vi "VisualizePurePursuit.vi"(7 "Lookahead Point":cluster{dbl, dbl}, 8 "Robot":cluster{"Location":cluster{dbl, dbl}, dbl}, 9 "Lookahead":dbl, 10 "Curvature":dbl, 11 "Path":cluster{"x":dbl, "y":dbl}[](array[cluster])=[{"x"=0.0, "y"=10.0}, {"x"=0.0, "y"=80.0}, {"x"=75.0, "y"=125.0}, {"x"=120.0, "y"=125.0}, {"x"=150.0, "y"=50.0}]) -> (3 "Graph":cluster{cluster{"x":dbl, "y":dbl}[]}[](graph)=[{[{"x"=0.0, "y"=10.0}, {"x"=3.061616997868383e-17, "y"=10.5}, {"x"=6.123233995736766e-17, "y"=11.0}, {"x"=9.184850993605148e-17, "y"=11.5}, {"x"=1.2246467991473532e-16, "y"=12.0}, {"x"=1.5308084989341916e-16, "y"=12.5}, {"x"=1.8369701987210297e-16, "y"=13.0}, {"x"=2.143131898507868e-16, "y"=13.5}, {"x"=2.4492935982947064e-16, "y"=14.0}, {"x"=2.755455298081545e-16, "y"=14.5}, {"x"=3.061616997868383e-16, "y"=15.0}, {"x"=3.3677786976552215e-16, "y"=15.5}, {"x"=3.6739403974420594e-16, "y"=16.0}, {"x"=3.9801020972288977e-16, "y"=16.5}, {"x"=4.286263797015736e-16, "y"=17.0}, {"x"=4.592425496802575e-16, "y"=17.5}, {"x"=4.898587196589413e-16, "y"=18.0}, {"x"=5.204748896376251e-16, "y"=18.5}, {"x"=5.51091059616309e-16, "y"=19.0}, {"x"=5.817072295949927e-16, "y"=19.5}, {"x"=6.123233995736766e-16, "y"=20.0}, {"x"=6.429395695523604e-16, "y"=20.5}, {"x"=6.735557395310443e-16, "y"=21.0}, {"x"=7.041719095097281e-16, "y"=21.5}, {"x"=7.347880794884119e-16, "y"=22.0}, {"x"=7.654042494670958e-16, "y"=22.5}, {"x"=7.960204194457795e-16, "y"=23.0}, {"x"=8.266365894244634e-16, "y"=23.5}, {"x"=8.572527594031472e-16, "y"=24.0}, {"x"=8.878689293818311e-16, "y"=24.5}, {"x"=9.18485099360515e-16, "y"=25.0}, {"x"=9.491012693391988e-16, "y"=25.5}, {"x"=9.797174393178826e-16, "y"=26.0}, {"x"=1.0103336092965664e-15, "y"=26.5}, {"x"=1.0409497792752501e-15, "y"=27.0}, {"x"=1.0715659492539341e-15, "y"=27.5}, {"x"=1.102182119232618e-15, "y"=28.0}, {"x"=1.1327982892113017e-15, "y"=28.5}, {"x"=1.1634144591899855e-15, "y"=29.0}, {"x"=1.1940306291686695e-15, "y"=29.5}, {"x"=1.2246467991473533e-15, "y"=30.0}, {"x"=1.255262969126037e-15, "y"=30.5}, {"x"=1.2858791391047208e-15, "y"=31.0}, {"x"=1.3164953090834046e-15, "y"=31.5}, {"x"=1.3471114790620886e-15, "y"=32.0}, {"x"=1.3777276490407724e-15, "y"=32.5}, {"x"=1.4083438190194562e-15, "y"=33.0}, {"x"=1.43895998899814e-15, "y"=33.5}, {"x"=1.4695761589768238e-15, "y"=34.0}, {"x"=1.5001923289555077e-15, "y"=34.5}, {"x"=1.5308084989341915e-15, "y"=35.0}, {"x"=1.5614246689128753e-15, "y"=35.5}, {"x"=1.592040838891559e-15, "y"=36.0}, {"x"=1.622657008870243e-15, "y"=36.5}, {"x"=1.6532731788489269e-15, "y"=37.0}, {"x"=1.6838893488276107e-15, "y"=37.5}, {"x"=1.7145055188062944e-15, "y"=38.0}, {"x"=1.7451216887849782e-15, "y"=38.5}, {"x"=1.7757378587636622e-15, "y"=39.0}, {"x"=1.8063540287423458e-15, "y"=39.5}, {"x"=1.83697019872103e-15, "y"=40.0}, {"x"=1.8675863686997138e-15, "y"=40.5}, {"x"=1.8982025386783976e-15, "y"=41.0}, {"x"=1.9288187086570813e-15, "y"=41.5}, {"x"=1.959434878635765e-15, "y"=42.0}, {"x"=1.990051048614449e-15, "y"=42.5}, {"x"=2.0206672185931327e-15, "y"=43.0}, {"x"=2.0512833885718165e-15, "y"=43.5}, {"x"=2.0818995585505003e-15, "y"=44.0}, {"x"=2.1125157285291845e-15, "y"=44.5}, {"x"=2.1431318985078682e-15, "y"=45.0}, {"x"=2.173748068486552e-15, "y"=45.5}, {"x"=2.204364238465236e-15, "y"=46.0}, {"x"=2.2349804084439196e-15, "y"=46.5}, {"x"=2.2655965784226034e-15, "y"=47.0}, {"x"=2.296212748401287e-15, "y"=47.5}, {"x"=2.326828918379971e-15, "y"=48.0}, {"x"=2.3574450883586548e-15, "y"=48.5}, {"x"=2.388061258337339e-15, "y"=49.0}, {"x"=2.4186774283160227e-15, "y"=49.5}, {"x"=2.4492935982947065e-15, "y"=50.0}, {"x"=2.4799097682733903e-15, "y"=50.5}, {"x"=2.510525938252074e-15, "y"=51.0}, {"x"=2.541142108230758e-15, "y"=51.5}, {"x"=2.5717582782094417e-15, "y"=52.0}, {"x"=2.6023744481881254e-15, "y"=52.5}, {"x"=2.6329906181668092e-15, "y"=53.0}, {"x"=2.6636067881454934e-15, "y"=53.5}, {"x"=2.6942229581241772e-15, "y"=54.0}, {"x"=2.724839128102861e-15, "y"=54.5}, {"x"=2.7554552980815448e-15, "y"=55.0}, {"x"=2.7860714680602286e-15, "y"=55.5}, {"x"=2.8166876380389124e-15, "y"=56.0}, {"x"=2.847303808017596e-15, "y"=56.5}, {"x"=2.87791997799628e-15, "y"=57.0}, {"x"=2.9085361479749637e-15, "y"=57.5}, {"x"=2.9391523179536475e-15, "y"=58.0}, {"x"=2.9697684879323317e-15, "y"=58.5}, {"x"=3.0003846579110155e-15, "y"=59.0}, {"x"=3.0310008278896993e-15, "y"=59.5}, {"x"=3.061616997868383e-15, "y"=60.0}, {"x"=3.092233167847067e-15, "y"=60.5}, {"x"=3.1228493378257506e-15, "y"=61.0}, {"x"=3.1534655078044344e-15, "y"=61.5}, {"x"=3.184081677783118e-15, "y"=62.0}, {"x"=3.214697847761802e-15, "y"=62.5}, {"x"=3.245314017740486e-15, "y"=63.0}, {"x"=3.27593018771917e-15, "y"=63.5}, {"x"=3.3065463576978537e-15, "y"=64.0}, {"x"=3.3371625276765375e-15, "y"=64.5}, {"x"=3.3677786976552213e-15, "y"=65.0}, {"x"=3.398394867633905e-15, "y"=65.5}, {"x"=3.429011037612589e-15, "y"=66.0}, {"x"=3.4596272075912727e-15, "y"=66.5}, {"x"=3.4902433775699565e-15, "y"=67.0}, {"x"=3.5208595475486406e-15, "y"=67.5}, {"x"=3.5514757175273244e-15, "y"=68.0}, {"x"=3.582091887506008e-15, "y"=68.5}, {"x"=3.6127080574846916e-15, "y"=69.0}, {"x"=3.643324227463376e-15, "y"=69.5}, {"x"=3.67394039744206e-15, "y"=70.0}, {"x"=3.704556567420744e-15, "y"=70.5}, {"x"=3.7351727373994275e-15, "y"=71.0}, {"x"=3.765788907378111e-15, "y"=71.5}, {"x"=3.796405077356795e-15, "y"=72.0}, {"x"=3.827021247335479e-15, "y"=72.5}, {"x"=3.857637417314163e-15, "y"=73.0}, {"x"=3.8882535872928465e-15, "y"=73.5}, {"x"=3.91886975727153e-15, "y"=74.0}, {"x"=3.949485927250214e-15, "y"=74.5}, {"x"=3.980102097228898e-15, "y"=75.0}, {"x"=4.010718267207582e-15, "y"=75.5}, {"x"=4.0413344371862654e-15, "y"=76.0}, {"x"=4.071950607164949e-15, "y"=76.5}, {"x"=4.102566777143633e-15, "y"=77.0}, {"x"=4.133182947122317e-15, "y"=77.5}, {"x"=4.1637991171010006e-15, "y"=78.0}, {"x"=4.194415287079684e-15, "y"=78.5}, {"x"=4.225031457058369e-15, "y"=79.0}, {"x"=4.255647627037053e-15, "y"=79.5}, {"x"=0.0, "y"=80.0}, {"x"=0.4287464628562721, "y"=80.25724787771377}, {"x"=0.8574929257125442, "y"=80.51449575542753}, {"x"=1.2862393885688164, "y"=80.77174363314128}, {"x"=1.7149858514250884, "y"=81.02899151085505}, {"x"=2.1437323142813605, "y"=81.28623938856882}, {"x"=2.5724787771376327, "y"=81.54348726628258}, {"x"=3.0012252399939046, "y"=81.80073514399635}, {"x"=3.429971702850177, "y"=82.0579830217101}, {"x"=3.858718165706449, "y"=82.31523089942387}, {"x"=4.287464628562721, "y"=82.57247877713763}, {"x"=4.716211091418993, "y"=82.8297266548514}, {"x"=5.1449575542752655, "y"=83.08697453256516}, {"x"=5.573704017131537, "y"=83.34422241027892}, {"x"=6.002450479987809, "y"=83.60147028799268}, {"x"=6.431196942844082, "y"=83.85871816570645}, {"x"=6.859943405700354, "y"=84.11596604342022}, {"x"=7.2886898685566255, "y"=84.37321392113398}, {"x"=7.717436331412898, "y"=84.63046179884773}, {"x"=8.14618279426917, "y"=84.8877096765615}, {"x"=8.574929257125442, "y"=85.14495755427527}, {"x"=9.003675719981715, "y"=85.40220543198903}, {"x"=9.432422182837986, "y"=85.6594533097028}, {"x"=9.861168645694258, "y"=85.91670118741655}, {"x"=10.289915108550531, "y"=86.17394906513032}, {"x"=10.718661571406802, "y"=86.43119694284408}, {"x"=11.147408034263075, "y"=86.68844482055785}, {"x"=11.576154497119347, "y"=86.94569269827161}, {"x"=12.004900959975618, "y"=87.20294057598537}, {"x"=12.433647422831891, "y"=87.46018845369913}, {"x"=12.862393885688164, "y"=87.7174363314129}, {"x"=13.291140348544435, "y"=87.97468420912666}, {"x"=13.719886811400707, "y"=88.23193208684043}, {"x"=14.14863327425698, "y"=88.48917996455418}, {"x"=14.577379737113251, "y"=88.74642784226795}, {"x"=15.006126199969524, "y"=89.00367571998171}, {"x"=15.434872662825796, "y"=89.26092359769548}, {"x"=15.863619125682067, "y"=89.51817147540925}, {"x"=16.29236558853834, "y"=89.775419353123}, {"x"=16.721112051394613, "y"=90.03266723083676}, {"x"=17.149858514250884, "y"=90.28991510855053}, {"x"=17.578604977107155, "y"=90.5471629862643}, {"x"=18.00735143996343, "y"=90.80441086397806}, {"x"=18.4360979028197, "y"=91.06165874169182}, {"x"=18.86484436567597, "y"=91.31890661940558}, {"x"=19.293590828532245, "y"=91.57615449711935}, {"x"=19.722337291388516, "y"=91.83340237483311}, {"x"=20.151083754244787, "y"=92.09065025254688}, {"x"=20.579830217101062, "y"=92.34789813026063}, {"x"=21.008576679957333, "y"=92.6051460079744}, {"x"=21.437323142813604, "y"=92.86239388568816}, {"x"=21.86606960566988, "y"=93.11964176340193}, {"x"=22.29481606852615, "y"=93.3768896411157}, {"x"=22.72356253138242, "y"=93.63413751882945}, {"x"=23.152308994238695, "y"=93.89138539654321}, {"x"=23.581055457094966, "y"=94.14863327425698}, {"x"=24.009801919951236, "y"=94.40588115197075}, {"x"=24.43854838280751, "y"=94.66312902968451}, {"x"=24.867294845663782, "y"=94.92037690739826}, {"x"=25.296041308520053, "y"=95.17762478511203}, {"x"=25.724787771376327, "y"=95.4348726628258}, {"x"=26.1535342342326, "y"=95.69212054053956}, {"x"=26.58228069708887, "y"=95.94936841825333}, {"x"=27.011027159945144, "y"=96.20661629596708}, {"x"=27.439773622801415, "y"=96.46386417368085}, {"x"=27.868520085657686, "y"=96.72111205139461}, {"x"=28.29726654851396, "y"=96.97835992910838}, {"x"=28.72601301137023, "y"=97.23560780682214}, {"x"=29.154759474226502, "y"=97.4928556845359}, {"x"=29.583505937082776, "y"=97.75010356224966}, {"x"=30.012252399939047, "y"=98.00735143996343}, {"x"=30.44099886279532, "y"=98.2645993176772}, {"x"=30.869745325651593, "y"=98.52184719539096}, {"x"=31.298491788507864, "y"=98.77909507310471}, {"x"=31.727238251364135, "y"=99.03634295081848}, {"x"=32.15598471422041, "y"=99.29359082853225}, {"x"=32.58473117707668, "y"=99.55083870624601}, {"x"=33.01347763993295, "y"=99.80808658395978}, {"x"=33.442224102789226, "y"=100.06533446167353}, {"x"=33.87097056564549, "y"=100.3225823393873}, {"x"=34.29971702850177, "y"=100.57983021710106}, {"x"=34.72846349135804, "y"=100.83707809481483}, {"x"=35.15720995421431, "y"=101.0943259725286}, {"x"=35.585956417070584, "y"=101.35157385024235}, {"x"=36.01470287992686, "y"=101.60882172795611}, {"x"=36.443449342783126, "y"=101.86606960566988}, {"x"=36.8721958056394, "y"=102.12331748338364}, {"x"=37.300942268495675, "y"=102.38056536109741}, {"x"=37.72968873135194, "y"=102.63781323881116}, {"x"=38.15843519420822, "y"=102.89506111652493}, {"x"=38.58718165706449, "y"=103.1523089942387}, {"x"=39.01592811992076, "y"=103.40955687195246}, {"x"=39.44467458277703, "y"=103.66680474966623}, {"x"=39.87342104563331, "y"=103.92405262737998}, {"x"=40.302167508489575, "y"=104.18130050509374}, {"x"=40.73091397134585, "y"=104.43854838280751}, {"x"=41.159660434202124, "y"=104.69579626052128}, {"x"=41.58840689705839, "y"=104.95304413823504}, {"x"=42.017153359914666, "y"=105.2102920159488}, {"x"=42.44589982277094, "y"=105.46753989366256}, {"x"=42.87464628562721, "y"=105.72478777137633}, {"x"=43.30339274848348, "y"=105.9820356490901}, {"x"=43.73213921133976, "y"=106.23928352680386}, {"x"=44.160885674196024, "y"=106.49653140451761}, {"x"=44.5896321370523, "y"=106.75377928223138}, {"x"=45.01837859990857, "y"=107.01102715994514}, {"x"=45.44712506276484, "y"=107.26827503765891}, {"x"=45.875871525621115, "y"=107.52552291537268}, {"x"=46.30461798847739, "y"=107.78277079308643}, {"x"=46.73336445133366, "y"=108.0400186708002}, {"x"=47.16211091418993, "y"=108.29726654851396}, {"x"=47.590857377046206, "y"=108.55451442622773}, {"x"=48.01960383990247, "y"=108.81176230394149}, {"x"=48.44835030275875, "y"=109.06901018165524}, {"x"=48.87709676561502, "y"=109.32625805936901}, {"x"=49.30584322847129, "y"=109.58350593708278}, {"x"=49.734589691327564, "y"=109.84075381479654}, {"x"=50.16333615418384, "y"=110.09800169251031}, {"x"=50.592082617040106, "y"=110.35524957022406}, {"x"=51.02082907989638, "y"=110.61249744793783}, {"x"=51.449575542752655, "y"=110.86974532565159}, {"x"=51.87832200560892, "y"=111.12699320336536}, {"x"=52.3070684684652, "y"=111.38424108107913}, {"x"=52.73581493132147, "y"=111.64148895879288}, {"x"=53.16456139417774, "y"=111.89873683650664}, {"x"=53.59330785703401, "y"=112.15598471422041}, {"x"=54.02205431989029, "y"=112.41323259193418}, {"x"=54.450800782746555, "y"=112.67048046964794}, {"x"=54.87954724560283, "y"=112.9277283473617}, {"x"=55.308293708459104, "y"=113.18497622507547}, {"x"=55.73704017131537, "y"=113.44222410278923}, {"x"=56.165786634171646, "y"=113.69947198050299}, {"x"=56.59453309702792, "y"=113.95671985821676}, {"x"=57.02327955988419, "y"=114.21396773593051}, {"x"=57.45202602274046, "y"=114.47121561364429}, {"x"=57.88077248559674, "y"=114.72846349135804}, {"x"=58.309518948453004, "y"=114.98571136907181}, {"x"=58.73826541130928, "y"=115.24295924678557}, {"x"=59.16701187416555, "y"=115.50020712449933}, {"x"=59.59575833702182, "y"=115.7574550022131}, {"x"=60.024504799878095, "y"=116.01470287992686}, {"x"=60.45325126273437, "y"=116.27195075764062}, {"x"=60.88199772559064, "y"=116.52919863535439}, {"x"=61.31074418844691, "y"=116.78644651306814}, {"x"=61.739490651303186, "y"=117.04369439078192}, {"x"=62.16823711415945, "y"=117.30094226849567}, {"x"=62.59698357701573, "y"=117.55819014620944}, {"x"=63.025730039872, "y"=117.8154380239232}, {"x"=63.45447650272827, "y"=118.07268590163696}, {"x"=63.883222965584544, "y"=118.32993377935074}, {"x"=64.31196942844082, "y"=118.58718165706449}, {"x"=64.74071589129709, "y"=118.84442953477826}, {"x"=65.16946235415335, "y"=119.10167741249202}, {"x"=65.59820881700963, "y"=119.35892529020578}, {"x"=66.0269552798659, "y"=119.61617316791956}, {"x"=66.45570174272217, "y"=119.87342104563331}, {"x"=66.88444820557845, "y"=120.13066892334707}, {"x"=67.31319466843472, "y"=120.38791680106084}, {"x"=67.74194113129099, "y"=120.64516467877459}, {"x"=68.17068759414727, "y"=120.90241255648837}, {"x"=68.59943405700353, "y"=121.15966043420212}, {"x"=69.0281805198598, "y"=121.41690831191589}, {"x"=69.45692698271608, "y"=121.67415618962966}, {"x"=69.88567344557235, "y"=121.93140406734341}, {"x"=70.31441990842862, "y"=122.18865194505719}, {"x"=70.7431663712849, "y"=122.44589982277094}, {"x"=71.17191283414117, "y"=122.7031477004847}, {"x"=71.60065929699743, "y"=122.96039557819847}, {"x"=72.02940575985372, "y"=123.21764345591222}, {"x"=72.45815222270998, "y"=123.474891333626}, {"x"=72.88689868556625, "y"=123.73213921133976}, {"x"=73.31564514842253, "y"=123.98938708905352}, {"x"=73.7443916112788, "y"=124.24663496676729}, {"x"=74.17313807413507, "y"=124.50388284448104}, {"x"=74.60188453699135, "y"=124.76113072219482}, {"x"=75.0, "y"=125.0}, {"x"=75.5, "y"=125.0}, {"x"=76.0, "y"=125.0}, {"x"=76.5, "y"=125.0}, {"x"=77.0, "y"=125.0}, {"x"=77.5, "y"=125.0}, {"x"=78.0, "y"=125.0}, {"x"=78.5, "y"=125.0}, {"x"=79.0, "y"=125.0}, {"x"=79.5, "y"=125.0}, {"x"=80.0, "y"=125.0}, {"x"=80.5, "y"=125.0}, {"x"=81.0, "y"=125.0}, {"x"=81.5, "y"=125.0}, {"x"=82.0, "y"=125.0}, {"x"=82.5, "y"=125.0}, {"x"=83.0, "y"=125.0}, {"x"=83.5, "y"=125.0}, {"x"=84.0, "y"=125.0}, {"x"=84.5, "y"=125.0}, {"x"=85.0, "y"=125.0}, {"x"=85.5, "y"=125.0}, {"x"=86.0, "y"=125.0}, {"x"=86.5, "y"=125.0}, {"x"=87.0, "y"=125.0}, {"x"=87.5, "y"=125.0}, {"x"=88.0, "y"=125.0}, {"x"=88.5, "y"=125.0}, {"x"=89.0, "y"=125.0}, {"x"=89.5, "y"=125.0}, {"x"=90.0, "y"=125.0}, {"x"=90.5, "y"=125.0}, {"x"=91.0, "y"=125.0}, {"x"=91.5, "y"=125.0}, {"x"=92.0, "y"=125.0}, {"x"=92.5, "y"=125.0}, {"x"=93.0, "y"=125.0}, {"x"=93.5, "y"=125.0}, {"x"=94.0, "y"=125.0}, {"x"=94.5, "y"=125.0}, {"x"=95.0, "y"=125.0}, {"x"=95.5, "y"=125.0}, {"x"=96.0, "y"=125.0}, {"x"=96.5, "y"=125.0}, {"x"=97.0, "y"=125.0}, {"x"=97.5, "y"=125.0}, {"x"=98.0, "y"=125.0}, {"x"=98.5, "y"=125.0}, {"x"=99.0, "y"=125.0}, {"x"=99.5, "y"=125.0}, {"x"=100.0, "y"=125.0}, {"x"=100.5, "y"=125.0}, {"x"=101.0, "y"=125.0}, {"x"=101.5, "y"=125.0}, {"x"=102.0, "y"=125.0}, {"x"=102.5, "y"=125.0}, {"x"=103.0, "y"=125.0}, {"x"=103.5, "y"=125.0}, {"x"=104.0, "y"=125.0}, {"x"=104.5, "y"=125.0}, {"x"=105.0, "y"=125.0}, {"x"=105.5, "y"=125.0}, {"x"=106.0, "y"=125.0}, {"x"=106.5, "y"=125.0}, {"x"=107.0, "y"=125.0}, {"x"=107.5, "y"=125.0}, {"x"=108.0, "y"=125.0}, {"x"=108.5, "y"=125.0}, {"x"=109.0, "y"=125.0}, {"x"=109.5, "y"=125.0}, {"x"=110.0, "y"=125.0}, {"x"=110.5, "y"=125.0}, {"x"=111.0, "y"=125.0}, {"x"=111.5, "y"=125.0}, {"x"=112.0, "y"=125.0}, {"x"=112.5, "y"=125.0}, {"x"=113.0, "y"=125.0}, {"x"=113.5, "y"=125.0}, {"x"=114.0, "y"=125.0}, {"x"=114.5, "y"=125.0}, {"x"=115.0, "y"=125.0}, {"x"=115.5, "y"=125.0}, {"x"=116.0, "y"=125.0}, {"x"=116.5, "y"=125.0}, {"x"=117.0, "y"=125.0}, {"x"=117.5, "y"=125.0}, {"x"=118.0, "y"=125.0}, {"x"=118.5, "y"=125.0}, {"x"=119.0, "y"=125.0}, {"x"=119.5, "y"=125.0}, {"x"=120.0, "y"=125.0}, {"x"=120.18569533817706, "y"=124.53576165455738}, {"x"=120.37139067635411, "y"=124.07152330911474}, {"x"=120.55708601453115, "y"=123.60728496367211}, {"x"=120.7427813527082, "y"=123.14304661822948}, {"x"=120.92847669088526, "y"=122.67880827278685}, {"x"=121.11417202906232, "y"=122.21456992734423}, {"x"=121.29986736723936, "y"=121.75033158190159}, {"x"=121.48556270541641, "y"=121.28609323645897}, {"x"=121.67125804359347, "y"=120.82185489101633}, {"x"=121.85695338177052, "y"=120.3576165455737}, {"x"=122.04264871994756, "y"=119.89337820013107}, {"x"=122.22834405812462, "y"=119.42913985468844}, {"x"=122.41403939630167, "y"=118.96490150924582}, {"x"=122.59973473447873, "y"=118.50066316380318}, {"x"=122.78543007265577, "y"=118.03642481836056}, {"x"=122.97112541083283, "y"=117.57218647291792}, {"x"=123.15682074900988, "y"=117.1079481274753}, {"x"=123.34251608718694, "y"=116.64370978203266}, {"x"=123.52821142536399, "y"=116.17947143659003}, {"x"=123.71390676354103, "y"=115.71523309114741}, {"x"=123.89960210171809, "y"=115.25099474570477}, {"x"=124.08529743989514, "y"=114.78675640026215}, {"x"=124.2709927780722, "y"=114.32251805481951}, {"x"=124.45668811624924, "y"=113.85827970937689}, {"x"=124.6423834544263, "y"=113.39404136393426}, {"x"=124.82807879260335, "y"=112.92980301849163}, {"x"=125.0137741307804, "y"=112.465564673049}, {"x"=125.19946946895746, "y"=112.00132632760636}, {"x"=125.3851648071345, "y"=111.53708798216374}, {"x"=125.57086014531156, "y"=111.07284963672112}, {"x"=125.75655548348861, "y"=110.60861129127848}, {"x"=125.94225082166567, "y"=110.14437294583585}, {"x"=126.12794615984271, "y"=109.68013460039322}, {"x"=126.31364149801976, "y"=109.2158962549506}, {"x"=126.49933683619682, "y"=108.75165790950797}, {"x"=126.68503217437387, "y"=108.28741956406533}, {"x"=126.87072751255091, "y"=107.82318121862271}, {"x"=127.05642285072797, "y"=107.35894287318007}, {"x"=127.24211818890502, "y"=106.89470452773745}, {"x"=127.42781352708208, "y"=106.43046618229482}, {"x"=127.61350886525912, "y"=105.96622783685218}, {"x"=127.79920420343618, "y"=105.50198949140955}, {"x"=127.98489954161323, "y"=105.03775114596692}, {"x"=128.1705948797903, "y"=104.5735128005243}, {"x"=128.35629021796734, "y"=104.10927445508166}, {"x"=128.5419855561444, "y"=103.64503610963904}, {"x"=128.72768089432145, "y"=103.1807977641964}, {"x"=128.91337623249848, "y"=102.71655941875377}, {"x"=129.09907157067553, "y"=102.25232107331115}, {"x"=129.2847669088526, "y"=101.78808272786851}, {"x"=129.47046224702964, "y"=101.32384438242589}, {"x"=129.6561575852067, "y"=100.85960603698325}, {"x"=129.84185292338375, "y"=100.39536769154063}, {"x"=130.0275482615608, "y"=99.931129346098}, {"x"=130.21324359973786, "y"=99.46689100065537}, {"x"=130.39893893791492, "y"=99.00265265521274}, {"x"=130.58463427609195, "y"=98.5384143097701}, {"x"=130.770329614269, "y"=98.07417596432748}, {"x"=130.95602495244606, "y"=97.60993761888486}, {"x"=131.1417202906231, "y"=97.14569927344222}, {"x"=131.32741562880017, "y"=96.6814609279996}, {"x"=131.51311096697722, "y"=96.21722258255696}, {"x"=131.69880630515428, "y"=95.75298423711433}, {"x"=131.88450164333133, "y"=95.28874589167171}, {"x"=132.07019698150836, "y"=94.82450754622907}, {"x"=132.25589231968542, "y"=94.36026920078645}, {"x"=132.44158765786247, "y"=93.89603085534381}, {"x"=132.62728299603953, "y"=93.43179250990119}, {"x"=132.81297833421658, "y"=92.96755416445856}, {"x"=132.99867367239364, "y"=92.50331581901592}, {"x"=133.1843690105707, "y"=92.03907747357329}, {"x"=133.37006434874775, "y"=91.57483912813066}, {"x"=133.55575968692477, "y"=91.11060078268804}, {"x"=133.74145502510183, "y"=90.64636243724541}, {"x"=133.92715036327888, "y"=90.18212409180278}, {"x"=134.11284570145594, "y"=89.71788574636014}, {"x"=134.298541039633, "y"=89.25364740091752}, {"x"=134.48423637781005, "y"=88.78940905547489}, {"x"=134.6699317159871, "y"=88.32517071003227}, {"x"=134.85562705416416, "y"=87.86093236458963}, {"x"=135.04132239234121, "y"=87.39669401914699}, {"x"=135.22701773051824, "y"=86.93245567370437}, {"x"=135.4127130686953, "y"=86.46821732826174}, {"x"=135.59840840687235, "y"=86.0039789828191}, {"x"=135.7841037450494, "y"=85.53974063737648}, {"x"=135.96979908322646, "y"=85.07550229193384}, {"x"=136.15549442140352, "y"=84.61126394649122}, {"x"=136.34118975958057, "y"=84.1470256010486}, {"x"=136.52688509775763, "y"=83.68278725560596}, {"x"=136.71258043593468, "y"=83.21854891016332}, {"x"=136.8982757741117, "y"=82.7543105647207}, {"x"=137.08397111228876, "y"=82.29007221927807}, {"x"=137.26966645046582, "y"=81.82583387383545}, {"x"=137.45536178864288, "y"=81.36159552839281}, {"x"=137.64105712681993, "y"=80.89735718295017}, {"x"=137.82675246499699, "y"=80.43311883750755}, {"x"=138.01244780317404, "y"=79.96888049206493}, {"x"=138.1981431413511, "y"=79.5046421466223}, {"x"=138.38383847952815, "y"=79.04040380117966}, {"x"=138.56953381770518, "y"=78.57616545573703}, {"x"=138.75522915588223, "y"=78.1119271102944}, {"x"=138.9409244940593, "y"=77.64768876485178}, {"x"=139.12661983223634, "y"=77.18345041940916}, {"x"=139.3123151704134, "y"=76.71921207396652}, {"x"=139.49801050859045, "y"=76.25497372852388}, {"x"=139.6837058467675, "y"=75.79073538308126}, {"x"=139.86940118494456, "y"=75.32649703763863}, {"x"=140.05509652312162, "y"=74.86225869219601}, {"x"=140.24079186129865, "y"=74.39802034675337}, {"x"=140.4264871994757, "y"=73.93378200131073}, {"x"=140.61218253765276, "y"=73.46954365586811}, {"x"=140.7978778758298, "y"=73.00530531042548}, {"x"=140.98357321400687, "y"=72.54106696498285}, {"x"=141.16926855218392, "y"=72.07682861954022}, {"x"=141.35496389036098, "y"=71.61259027409758}, {"x"=141.540659228538, "y"=71.14835192865496}, {"x"=141.72635456671506, "y"=70.68411358321234}, {"x"=141.91204990489211, "y"=70.2198752377697}, {"x"=142.09774524306917, "y"=69.75563689232706}, {"x"=142.28344058124623, "y"=69.29139854688444}, {"x"=142.46913591942328, "y"=68.82716020144181}, {"x"=142.65483125760034, "y"=68.36292185599919}, {"x"=142.8405265957774, "y"=67.89868351055655}, {"x"=143.02622193395445, "y"=67.43444516511391}, {"x"=143.21191727213147, "y"=66.97020681967129}, {"x"=143.39761261030853, "y"=66.50596847422867}, {"x"=143.58330794848558, "y"=66.04173012878604}, {"x"=143.76900328666264, "y"=65.5774917833434}, {"x"=143.9546986248397, "y"=65.11325343790077}, {"x"=144.14039396301675, "y"=64.64901509245814}, {"x"=144.3260893011938, "y"=64.18477674701552}, {"x"=144.51178463937086, "y"=63.72053840157289}, {"x"=144.6974799775479, "y"=63.25630005613026}, {"x"=144.88317531572494, "y"=62.792061710687626}, {"x"=145.068870653902, "y"=62.327823365244996}, {"x"=145.25456599207905, "y"=61.863585019802365}, {"x"=145.4402613302561, "y"=61.39934667435974}, {"x"=145.62595666843316, "y"=60.93510832891711}, {"x"=145.81165200661022, "y"=60.47086998347447}, {"x"=145.99734734478727, "y"=60.00663163803185}, {"x"=146.18304268296433, "y"=59.542393292589225}, {"x"=146.36873802114138, "y"=59.07815494714659}, {"x"=146.5544333593184, "y"=58.61391660170396}, {"x"=146.74012869749546, "y"=58.149678256261325}, {"x"=146.92582403567252, "y"=57.6854399108187}, {"x"=147.11151937384957, "y"=57.22120156537608}, {"x"=147.29721471202663, "y"=56.75696321993344}, {"x"=147.48291005020369, "y"=56.292724874490816}, {"x"=147.66860538838074, "y"=55.82848652904818}, {"x"=147.8543007265578, "y"=55.364248183605554}, {"x"=148.03999606473485, "y"=54.900009838162916}, {"x"=148.22569140291188, "y"=54.43577149272029}, {"x"=148.41138674108893, "y"=53.97153314727767}, {"x"=148.597082079266, "y"=53.50729480183503}, {"x"=148.78277741744304, "y"=53.04305645639241}, {"x"=148.9684727556201, "y"=52.57881811094977}, {"x"=149.15416809379715, "y"=52.114579765507145}, {"x"=149.3398634319742, "y"=51.65034142006452}, {"x"=149.52555877015124, "y"=51.18610307462188}, {"x"=149.7112541083283, "y"=50.72186472917926}, {"x"=149.89694944650535, "y"=50.25762638373662}, {"x"=150.0, "y"=50.0}]}, {[{"x"=131.14560801363658, "y"=98.05139678064754}, {"x"=134.38374214186317, "y"=88.59018716624757}]}, {[{"x"=138.1981431413511, "y"=79.5046421466223}]}, {[{"x"=151.14560801363658, "y"=98.05139678064754}, {"x"=151.106142582202, "y"=99.3072071712338}, {"x"=150.98790203992613, "y"=100.55806145193363}, {"x"=150.79135302821035, "y"=101.79902307236203}, {"x"=150.51727123620918, "y"=103.02519452394463}, {"x"=150.16673833953965, "y"=104.23173666814648}, {"x"=149.7411377314016, "y"=105.4138878343411}, {"x"=149.24214906295697, "y"=106.56698261194899}, {"x"=148.67174161451385, "y"=107.68647026268184}, {"x"=148.0321665236769, "y"=108.76793268022747}, {"x"=147.32594790113552, "y"=109.807101826497}, {"x"=146.55587286915235, "y"=110.79987657562133}, {"x"=145.72498056206481, "y"=111.74233889922131}, {"x"=144.83655013221033, "y"=112.63076932907578}, {"x"=143.89408780861038, "y"=113.46166163616331}, {"x"=142.90131305948603, "y"=114.23173666814648}, {"x"=141.8621439132165, "y"=114.93795529068784}, {"x"=140.78068149567088, "y"=115.57753038152481}, {"x"=139.66119384493803, "y"=116.14793782996793}, {"x"=138.50809906733014, "y"=116.64692649841257}, {"x"=137.32594790113552, "y"=117.07252710655061}, {"x"=136.11940575693367, "y"=117.42306000322016}, {"x"=134.89323430535106, "y"=117.69714179522131}, {"x"=133.65227268492265, "y"=117.89369080693709}, {"x"=132.40141840422285, "y"=118.01193134921297}, {"x"=131.14560801363658, "y"=118.05139678064754}, {"x"=129.8897976230503, "y"=118.01193134921297}, {"x"=128.6389433423505, "y"=117.89369080693709}, {"x"=127.39798172192208, "y"=117.69714179522131}, {"x"=126.17181027033948, "y"=117.42306000322016}, {"x"=124.96526812613763, "y"=117.07252710655061}, {"x"=123.78311695994302, "y"=116.64692649841257}, {"x"=122.63002218233513, "y"=116.14793782996793}, {"x"=121.51053453160227, "y"=115.57753038152481}, {"x"=120.42907211405664, "y"=114.93795529068784}, {"x"=119.38990296778712, "y"=114.23173666814648}, {"x"=118.39712821866279, "y"=113.46166163616331}, {"x"=117.4546658950628, "y"=112.63076932907576}, {"x"=116.56623546520834, "y"=111.74233889922131}, {"x"=115.73534315812078, "y"=110.79987657562133}, {"x"=114.96526812613763, "y"=109.807101826497}, {"x"=114.25904950359627, "y"=108.76793268022747}, {"x"=113.6194744127593, "y"=107.68647026268184}, {"x"=113.04906696431618, "y"=106.56698261194899}, {"x"=112.55007829587154, "y"=105.4138878343411}, {"x"=112.1244776877335, "y"=104.23173666814648}, {"x"=111.77394479106395, "y"=103.02519452394463}, {"x"=111.4998629990628, "y"=101.79902307236203}, {"x"=111.30331398734702, "y"=100.55806145193361}, {"x"=111.18507344507114, "y"=99.3072071712338}, {"x"=111.14560801363658, "y"=98.05139678064754}, {"x"=111.18507344507114, "y"=96.79558639006127}, {"x"=111.30331398734702, "y"=95.54473210936145}, {"x"=111.4998629990628, "y"=94.30377048893304}, {"x"=111.77394479106395, "y"=93.07759903735044}, {"x"=112.1244776877335, "y"=91.87105689314858}, {"x"=112.55007829587154, "y"=90.68890572695398}, {"x"=113.04906696431618, "y"=89.53581094934609}, {"x"=113.6194744127593, "y"=88.41632329861324}, {"x"=114.25904950359627, "y"=87.3348608810676}, {"x"=114.96526812613763, "y"=86.29569173479807}, {"x"=115.7353431581208, "y"=85.30291698567373}, {"x"=116.56623546520834, "y"=84.36045466207376}, {"x"=117.4546658950628, "y"=83.4720242322193}, {"x"=118.39712821866279, "y"=82.64113192513175}, {"x"=119.38990296778711, "y"=81.87105689314859}, {"x"=120.42907211405665, "y"=81.16483827060723}, {"x"=121.51053453160227, "y"=80.52526317977026}, {"x"=122.63002218233513, "y"=79.95485573132714}, {"x"=123.78311695994302, "y"=79.4558670628825}, {"x"=124.96526812613763, "y"=79.03026645474446}, {"x"=126.17181027033949, "y"=78.67973355807491}, {"x"=127.39798172192208, "y"=78.40565176607376}, {"x"=128.6389433423505, "y"=78.20910275435799}, {"x"=129.8897976230503, "y"=78.0908622120821}, {"x"=131.14560801363658, "y"=78.05139678064754}, {"x"=132.40141840422285, "y"=78.0908622120821}, {"x"=133.65227268492265, "y"=78.20910275435799}, {"x"=134.8932343053511, "y"=78.40565176607376}, {"x"=136.11940575693367, "y"=78.67973355807491}, {"x"=137.32594790113552, "y"=79.03026645474446}, {"x"=138.50809906733014, "y"=79.4558670628825}, {"x"=139.66119384493803, "y"=79.95485573132714}, {"x"=140.78068149567088, "y"=80.52526317977026}, {"x"=141.8621439132165, "y"=81.16483827060723}, {"x"=142.90131305948606, "y"=81.87105689314859}, {"x"=143.89408780861038, "y"=82.64113192513176}, {"x"=144.83655013221033, "y"=83.4720242322193}, {"x"=145.72498056206481, "y"=84.36045466207378}, {"x"=146.55587286915235, "y"=85.30291698567375}, {"x"=147.32594790113552, "y"=86.29569173479808}, {"x"=148.0321665236769, "y"=87.33486088106761}, {"x"=148.67174161451385, "y"=88.41632329861324}, {"x"=149.24214906295697, "y"=89.53581094934609}, {"x"=149.7411377314016, "y"=90.68890572695398}, {"x"=150.16673833953965, "y"=91.8710568931486}, {"x"=150.5172712362092, "y"=93.07759903735045}, {"x"=150.79135302821035, "y"=94.30377048893304}, {"x"=150.98790203992613, "y"=95.54473210936146}, {"x"=151.106142582202, "y"=96.79558639006127}, {"x"=151.14560801363658, "y"=98.05139678064755}]}, {[{"x"=114.98666496898397, "y"=195.16676176750735}, {"x"=115.57847179760216, "y"=176.33516313591082}, {"x"=117.35155669227487, "y"=157.57788422077414}, {"x"=120.29892209696834, "y"=138.96895143258976}, {"x"=124.40893610695349, "y"=120.58180572745995}, {"x"=129.66537837461954, "y"=102.48901276919503}, {"x"=136.04750412377615, "y"=84.76197654579038}, {"x"=143.53012601980726, "y"=67.47065757050733}, {"x"=152.08371357257408, "y"=50.68329677968913}, {"x"=161.6745096797682, "y"=34.466146216961505}, {"x"=172.2646638507725, "y"=18.883207566684177}, {"x"=183.81238158525534, "y"=3.995979568542282}, {"x"=196.27208931696896, "y"=-10.136784689882973}, {"x"=209.59461427179545, "y"=-23.459309644709435}, {"x"=223.7273785302207, "y"=-35.919017376423085}, {"x"=238.6146065283626, "y"=-47.46673511090589}, {"x"=254.19754517863993, "y"=-58.0568892819102}, {"x"=270.4146957413676, "y"=-67.64768538910437}, {"x"=287.20205653218574, "y"=-76.20127294187114}, {"x"=304.49337550746884, "y"=-83.6838948379023}, {"x"=322.22041173087337, "y"=-90.06602058705886}, {"x"=340.3132046891384, "y"=-95.3224628547249}, {"x"=358.7003503942682, "y"=-99.43247686471005}, {"x"=377.30928318245253, "y"=-102.37984226940353}, {"x"=396.0665620975892, "y"=-104.15292716407623}, {"x"=414.8981607291858, "y"=-104.74473399269442}, {"x"=433.7297593607823, "y"=-104.15292716407623}, {"x"=452.487038275919, "y"=-102.37984226940347}, {"x"=471.0959710641034, "y"=-99.43247686471}, {"x"=489.48311676923316, "y"=-95.3224628547249}, {"x"=507.57590972749813, "y"=-90.06602058705886}, {"x"=525.3029459509028, "y"=-83.68389483790224}, {"x"=542.5942649261858, "y"=-76.20127294187114}, {"x"=559.381625717004, "y"=-67.64768538910431}, {"x"=575.5987762797317, "y"=-58.05688928191017}, {"x"=591.1817149300089, "y"=-47.46673511090589}, {"x"=606.0689429281508, "y"=-35.919017376423085}, {"x"=620.2017071865761, "y"=-23.45930964470938}, {"x"=633.5242321414025, "y"=-10.136784689882916}, {"x"=645.9839398731162, "y"=3.995979568542367}, {"x"=657.531657607599, "y"=18.88320756668412}, {"x"=668.1218117786033, "y"=34.466146216961505}, {"x"=677.7126078857974, "y"=50.68329677968916}, {"x"=686.2661954385642, "y"=67.4706575705074}, {"x"=693.7488173345954, "y"=84.76197654579045}, {"x"=700.1309430837521, "y"=102.4890127691951}, {"x"=705.3873853514181, "y"=120.58180572745994}, {"x"=709.4973993614032, "y"=138.9689514325898}, {"x"=712.4447647660966, "y"=157.5778842207742}, {"x"=714.2178496607694, "y"=176.33516313591088}, {"x"=714.8096564893875, "y"=195.16676176750744}, {"x"=714.2178496607694, "y"=213.9983603991039}, {"x"=712.4447647660966, "y"=232.75563931424057}, {"x"=709.497399361403, "y"=251.36457210242497}, {"x"=705.3873853514181, "y"=269.7517178075548}, {"x"=700.130943083752, "y"=287.8445107658198}, {"x"=693.7488173345953, "y"=305.57154698922443}, {"x"=686.2661954385642, "y"=322.86286596450736}, {"x"=677.7126078857974, "y"=339.6502267553256}, {"x"=668.1218117786033, "y"=355.8673773180533}, {"x"=657.5316576075988, "y"=371.45031596833064}, {"x"=645.9839398731161, "y"=386.3375439664725}, {"x"=633.5242321414025, "y"=400.4703082248977}, {"x"=620.2017071865761, "y"=413.79283317972414}, {"x"=606.0689429281507, "y"=426.2525409114378}, {"x"=591.181714930009, "y"=437.80025864592056}, {"x"=575.5987762797315, "y"=448.39041281692494}, {"x"=559.381625717004, "y"=457.981208924119}, {"x"=542.5942649261856, "y"=466.5347964768859}, {"x"=525.3029459509027, "y"=474.017418372917}, {"x"=507.57590972749813, "y"=480.39954412207356}, {"x"=489.48311676923305, "y"=485.65598638973967}, {"x"=471.0959710641033, "y"=489.76600039972476}, {"x"=452.4870382759188, "y"=492.71336580441823}, {"x"=433.7297593607822, "y"=494.48645069909094}, {"x"=414.8981607291858, "y"=495.0782575277091}, {"x"=396.0665620975891, "y"=494.48645069909094}, {"x"=377.30928318245253, "y"=492.71336580441823}, {"x"=358.700350394268, "y"=489.7660003997247}, {"x"=340.3132046891383, "y"=485.6559863897396}, {"x"=322.2204117308735, "y"=480.3995441220736}, {"x"=304.49337550746867, "y"=474.0174183729169}, {"x"=287.2020565321858, "y"=466.53479647688584}, {"x"=270.4146957413674, "y"=457.98120892411896}, {"x"=254.19754517863984, "y"=448.3904128169249}, {"x"=238.6146065283624, "y"=437.80025864592045}, {"x"=223.72737853022062, "y"=426.25254091143773}, {"x"=209.59461427179545, "y"=413.79283317972414}, {"x"=196.27208931696887, "y"=400.4703082248975}, {"x"=183.81238158525528, "y"=386.33754396647237}, {"x"=172.26466385077242, "y"=371.4503159683304}, {"x"=161.67450967976814, "y"=355.8673773180531}, {"x"=152.08371357257408, "y"=339.65022675532555}, {"x"=143.5301260198072, "y"=322.86286596450725}, {"x"=136.0475041237761, "y"=305.5715469892243}, {"x"=129.66537837461948, "y"=287.8445107658195}, {"x"=124.40893610695343, "y"=269.75171780755466}, {"x"=120.29892209696834, "y"=251.36457210242497}, {"x"=117.35155669227487, "y"=232.75563931424043}, {"x"=115.57847179760216, "y"=213.99836039910386}, {"x"=114.98666496898397, "y"=195.16676176750715}]}])   [LabVIEW 2016]
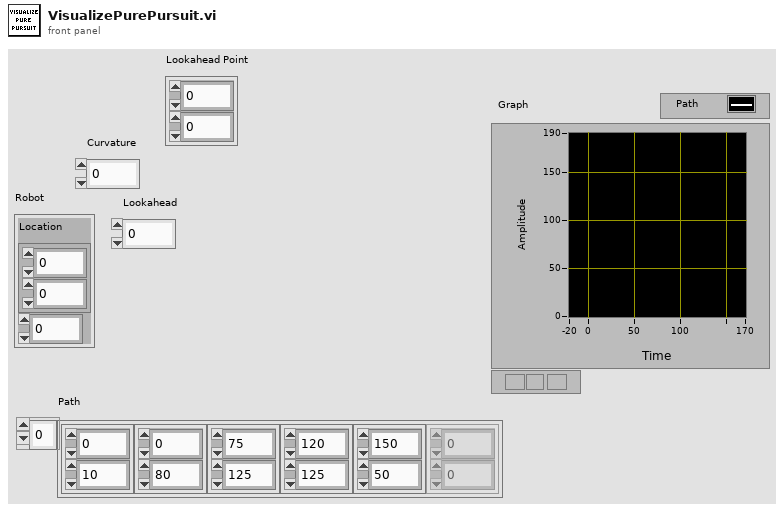
[diagram p1: front panel]
types:
  T1 = cluster{"Circle Graph":cluster{"x":dbl, "y":dbl}[]}[]
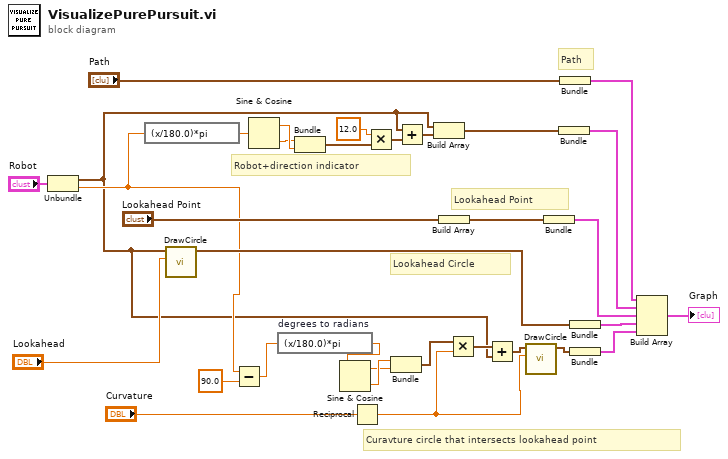
[diagram p0: block diagram]
diagram:
  # "Curavture circle that intersects lookahead point"
  # "Lookahead Circle"
  # "Lookahead Point"
  # "Robot+direction indicator"
  # "Path"
  n1 = Unbundle("Robot") -> ("Location"=w4:cluster{dbl, dbl}, w5:dbl)
  n2 = expression code="(x/180.0)*pi" ("degrees to radians")(w5) -> (w14:dbl)
  n3 = call "DrawCircle.vi"("r"="Lookahead", "Center"=w4) -> ("Circle Graph"=w8:cluster{dbl, dbl}[])  [unwired: 9 in]
  n4 = Subtract(x=w5, y=90.0) -> (x-y=w2:dbl)
  n5 = Sine & Cosine(0:w14) -> (1:w20:dbl, 2:w19:dbl)
  n6 = expression code="(x/180.0)*pi" "degrees to radians"(w2) -> (w1:dbl)
  n7 = Bundle(w19, w20) -> (w17:cluster{dbl, dbl})  [unwired: 1 in]
  n8 = Sine & Cosine(0:w1) -> (1:w30:dbl, 2:w31:dbl)
  n9 = Reciprocal(x="Curvature") -> (1/x=w25:dbl)
  n10 = Multiply(x=12.0 ("Angle"), y=w17) -> (x*y=w16:cluster{dbl, dbl})
  n11 = Bundle(w31, w30) -> (w29:cluster{dbl, dbl})  [unwired: 1 in]
  n12 = Add(x=w4, y=w16) -> (x+y=w18:cluster{dbl, dbl})
  n13 = Build Array(w4, w18) -> (w13:cluster{dbl, dbl}[])
  n14 = Build Array("Lookahead Point") -> (w11:cluster{dbl, dbl}[])
  n15 = Multiply(x=w29, y=w25) -> (x*y=w28:cluster{dbl, dbl})
  n16 = Add(x=w28, y=w4) -> (x+y=w26:cluster{dbl, dbl})
  n17 = call "DrawCircle.vi"("r"=w25, "Center"=w26) -> ("Circle Graph"=w24:cluster{dbl, dbl}[])  [unwired: 9 in]
  n18 = Bundle(w11) -> (w10:cluster{cluster{dbl, dbl}[]})  [unwired: 1 in]
  n19 = Bundle(w13) -> (w33:cluster{cluster{dbl, dbl}[]})  [unwired: 1 in]
  n20 = Bundle("Path"="Path") -> (w22:cluster{"Path":cluster{"x":dbl, "y":dbl}[]})  [unwired: 1 in]
  n21 = Bundle("Circle Graph"=w8) -> (w7:cluster{"Circle Graph":cluster{dbl, dbl}[]})  [unwired: 1 in]
  n22 = Bundle("Circle Graph"=w24) -> (w32:cluster{"Circle Graph":cluster{dbl, dbl}[]})  [unwired: 1 in]
  n23 = Build Array(w22, w33, w10, w7, w32) -> (→"Graph":T1)
